vi "Julabo_Get_All_Values_subVI.vi"(4 "Reset / Default (T: Both)":bool=TRUE, 6 "ID Query? (T: Yes)":bool=TRUE, 7 "Data Cluster In":T1={"Current DoE"=[], "SSI 1 Flow Rate"=0.0, "SSI 2 Flow Rate"=0.0, "FLOM 1 Flow Rate"=0.0, "FLOM 2 Flow Rate"=0.0, "Pumps Running?"=FALSE, "Boolean 2"=FALSE, "Boolean 3"=FALSE, "Boolean 4"=FALSE, "At Equilibrium?"=FALSE, "Script Running?"=FALSE, "Current Script Iteration"=0.0, "Total Script Iterations"=0.0, "FLOM Pumps VISA"="COM2", "SSI 1 Pump VISA"="COM76", "SSI 2 Pump VISA"="COM74", "Huber Unistat VISA"="COM1", "SSI 3 Pump VISA"="COM76", "SSI 4 Pump VISA"="COM76", "SSI 4 Flow Rate"=0.0, "SSI 3 Flow Rate"=0.0, "Flow Meter 1 Rate "=0.0, "Flow Meter 2 Rate"=0.0, "Flow Meter 3 Rate"=0.0, "Flow Meter 4 Rate"=0.0, "SSI 1 Flow Setpoint"=0.0, "SSI 2 Flow Setpoint"=0.0, "SSI 3 Flow Setpoint"=0.0, "SSI 4 Flow Setpoint"=0.0, "Temperature Setpoint"=0.0, "Flow meter 3 COM"=17, "Flow meter 5 COM"=18, "Flow meter 4 COM"=19, "Flow meter 2 COM"=16, "Flow meter 1 COM"=15, "Unit"=enum."PSI", "Pressure COM"="COM6", "Julabo Setpoint"=0.0, "Julabo Control"=enum."Internal", "Overtemp"=50.0, "Subtemp"=-20.0, "HeatMax"=50, "CoolMax"=-100, "InternMax"=50.0, "InternMin"=0.0, "Upper Bandlimit"=100.0, "Lower Bandlimit"=0.0, "Julabo CF41 VISA"="COM3", "Xp (0.6K) Int"=0.6, "Tn (3s) Int"=3, "Tv (0s) Int"=0, "Dynamic (0: aperiodic) Int"=enum."aperiodic", "Xp (0.6K) Ext"=0.6, "Tn (3s) Ext"=3, "Tv (0s) Ext"=0, "XpU (0.6K) Ext"=0.6} {"XpU (0.6K) Ext" min=0.1 max=99.9; "Tv (0s) Ext" max=999; "Tn (3s) Ext" min=3 max=9999; "Xp (0.6K) Ext" min=0.1 max=99.9; "Tv (0s) Int" max=999; "Tn (3s) Int" min=3 max=9999; "Xp (0.6K) Int" min=0.1 max=99.9; "Lower Bandlimit" min=0.0 max=200.0; "Upper Bandlimit" min=0.0 max=200.0; "InternMin" format="%.2f"; "InternMax" format="%.2f"; "CoolMax" min=-100 max=0; "HeatMax" max=100; "Subtemp" format="%.2f"; "Overtemp" format="%.2f"; "Julabo Setpoint" format="%.2f"; "Current DoE" format="%0.3f"}, 9 "Serial Configuration":T2={"Baud Rate"=4800, "Parity"=2, "Data Bits"=7, "Stop Bits"=10, "Flow Control"=2} {"Flow Control" items=["None", "XON/XOFF", "RTS/CTS", "XON/XOFF & RTS/CTS", "DTR/DSR", "XON/XOFF & DTR/DSR"]; "Stop Bits" items=["1.0"=10, "1.5"=15, "2.0"=20]; "Data Bits" items=["7"=7, "8"=8]; "Parity" items=["None", "Odd", "Even", "Mark", "Space"]; "Baud Rate" items=["300"=300, "600"=600, "1200"=1200, "2400"=2400, "4800"=4800, "9600"=9600, "19200"=19200]}, 10 "RS485-Address (128: RS232)":u32=128, 11 "VISA Refnum in":refnum<visa-resource-name>="COM3") -> (0 "error out":errorcluster, 2 "Setpointindex":enum16{"Setpoint 1", "Setpoint 2", "Setpoint 3"}(ring), 5 "Data Cluster Out":T1={"Current DoE"=[], "SSI 1 Flow Rate"=0.0, "SSI 2 Flow Rate"=0.0, "FLOM 1 Flow Rate"=0.0, "FLOM 2 Flow Rate"=0.0, "Pumps Running?"=FALSE, "Boolean 2"=FALSE, "Boolean 3"=FALSE, "Boolean 4"=FALSE, "At Equilibrium?"=FALSE, "Script Running?"=FALSE, "Current Script Iteration"=0.0, "Total Script Iterations"=0.0, "FLOM Pumps VISA"="COM2", "SSI 1 Pump VISA"="COM76", "SSI 2 Pump VISA"="COM74", "Huber Unistat VISA"="COM1", "SSI 3 Pump VISA"="COM76", "SSI 4 Pump VISA"="COM76", "SSI 4 Flow Rate"=0.0, "SSI 3 Flow Rate"=0.0, "Flow Meter 1 Rate "=0.0, "Flow Meter 2 Rate"=0.0, "Flow Meter 3 Rate"=0.0, "Flow Meter 4 Rate"=0.0, "SSI 1 Flow Setpoint"=0.0, "SSI 2 Flow Setpoint"=0.0, "SSI 3 Flow Setpoint"=0.0, "SSI 4 Flow Setpoint"=0.0, "Temperature Setpoint"=0.0, "Flow meter 3 COM"=17, "Flow meter 5 COM"=18, "Flow meter 4 COM"=19, "Flow meter 2 COM"=16, "Flow meter 1 COM"=15, "Unit"=enum."PSI", "Pressure COM"="COM6", "Julabo Setpoint"=0.0, "Julabo Control"=enum."Internal", "Overtemp"=50.0, "Subtemp"=-20.0, "HeatMax"=50, "CoolMax"=-100, "InternMax"=50.0, "InternMin"=0.0, "Upper Bandlimit"=100.0, "Lower Bandlimit"=0.0, "Julabo CF41 VISA"="COM3", "Xp (0.6K) Int"=0.6, "Tn (3s) Int"=3, "Tv (0s) Int"=0, "Dynamic (0: aperiodic) Int"=enum."aperiodic", "Xp (0.6K) Ext"=0.6, "Tn (3s) Ext"=3, "Tv (0s) Ext"=0, "XpU (0.6K) Ext"=0.6} {"XpU (0.6K) Ext" min=0.1 max=99.9; "Tv (0s) Ext" max=999; "Tn (3s) Ext" min=3 max=9999; "Xp (0.6K) Ext" min=0.1 max=99.9; "Tv (0s) Int" max=999; "Tn (3s) Int" min=3 max=9999; "Xp (0.6K) Int" min=0.1 max=99.9; "Lower Bandlimit" min=0.0 max=200.0; "Upper Bandlimit" min=0.0 max=200.0; "InternMin" format="%.2f"; "InternMax" format="%.2f"; "CoolMax" min=-100 max=0; "HeatMax" max=100; "Subtemp" format="%.2f"; "Overtemp" format="%.2f"; "Julabo Setpoint" format="%.2f"; "Current DoE" format="%0.3f"})   [LabVIEW 2015, in "JULABO DeviceDriver.lvlib"]
uses:
  <instrlib>/JULABO DeviceDriver/JULABO DeviceDriver.lvlib
  <instrlib>/JULABO DeviceDriver/Examples/Julabo Serial Control.ctl
  --Controls and TypeDefs--/DoE_Control_Cluster.ctl
panel:
  # "Julabo"
  # "Limits"
  # "PID Control Parameters"
  # "Julabo"
  # "Limits"
  # "PID Control Parameters"
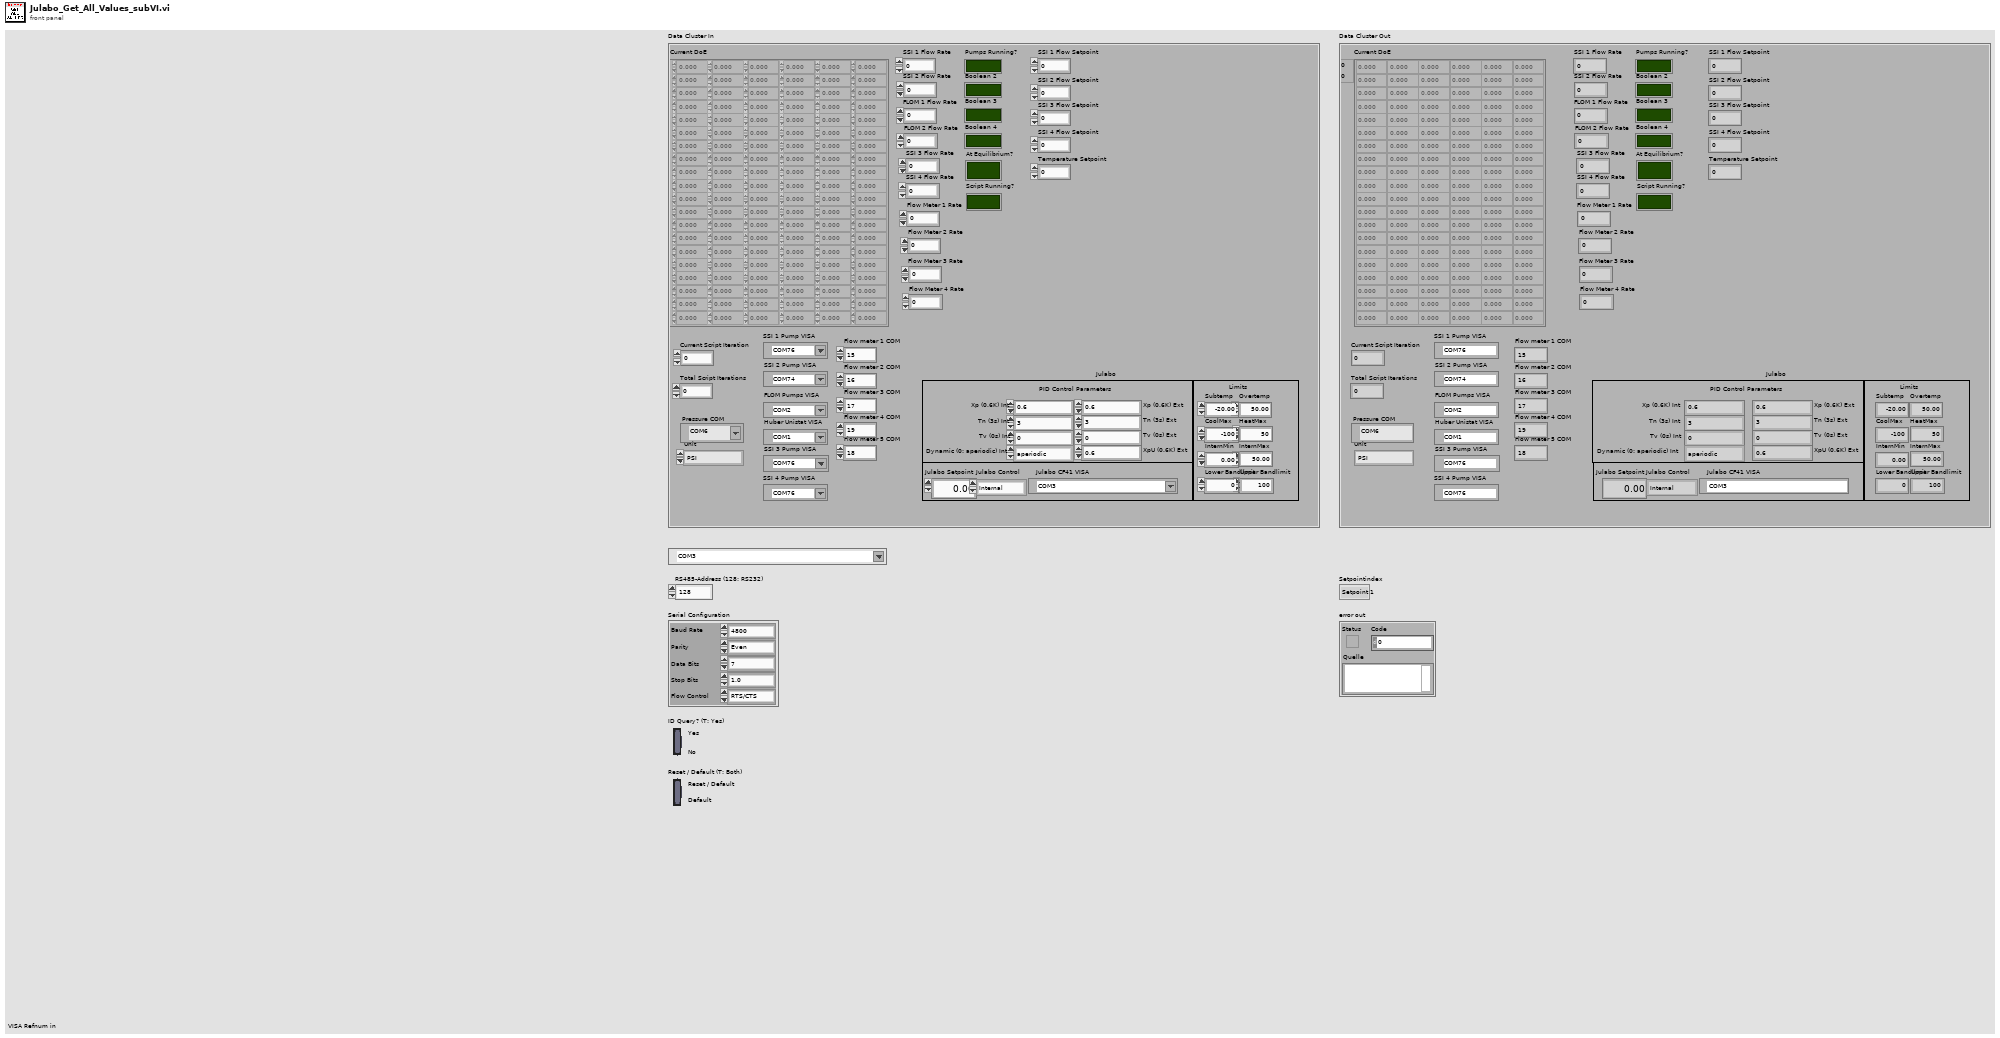
[diagram p1: front panel]
types:
  T1 = typedef "DoE_Control_Cluster.ctl" = cluster{"Current DoE":dbl[][], "SSI 1 Flow Rate":dbl, "SSI 2 Flow Rate":dbl, "FLOM 1 Flow Rate":dbl, "FLOM 2 Flow Rate":dbl, "Pumps Running?":bool, "Boolean 2":bool, "Boolean 3":bool, "Boolean 4":bool, "At Equilibrium?":bool, "Script Running?":bool, "Current Script Iteration":dbl, "Total Script Iterations":dbl, "FLOM Pumps VISA":refnum<visa-resource-name>, "SSI 1 Pump VISA":refnum<visa-resource-name>, "SSI 2 Pump VISA":refnum<visa-resource-name>, "Huber Unistat VISA":refnum<visa-resource-name>, "SSI 3 Pump VISA":refnum<visa-resource-name>, "SSI 4 Pump VISA":refnum<visa-resource-name>, "SSI 4 Flow Rate":dbl, "SSI 3 Flow Rate":dbl, "Flow Meter 1 Rate ":dbl, "Flow Meter 2 Rate":dbl, "Flow Meter 3 Rate":dbl, "Flow Meter 4 Rate":dbl, "SSI 1 Flow Setpoint":dbl, "SSI 2 Flow Setpoint":dbl, "SSI 3 Flow Setpoint":dbl, "SSI 4 Flow Setpoint":dbl, "Temperature Setpoint":dbl, "Flow meter 3 COM":u16, "Flow meter 5 COM":u16, "Flow meter 4 COM":u16, "Flow meter 2 COM":u16, "Flow meter 1 COM":u16, "Unit":enum16{"PSI", "Bar", "cm H2O", "ft H2O", "hectoPascal", "in Hg", "in H2O", "kiloPascal", "milliBar", "mmHg", "MegaPascal", "Numeric Pressure"}, "Pressure COM":refnum<visa-resource-name>, "Julabo Setpoint":dbl, "Julabo Control":enum16{"Internal", "External"}, "Overtemp":dbl, "Subtemp":dbl, "HeatMax":u8, "CoolMax":i8, "InternMax":dbl, "InternMin":dbl, "Upper Bandlimit":dbl, "Lower Bandlimit":dbl, "Julabo CF41 VISA":refnum<visa-resource-name>, "Xp (0.6K) Int":dbl, "Tn (3s) Int":u16, "Tv (0s) Int":u16, "Dynamic (0: aperiodic) Int":enum16{"aperiodic", "standard"}, "Xp (0.6K) Ext":dbl, "Tn (3s) Ext":u16, "Tv (0s) Ext":u16, "XpU (0.6K) Ext":dbl}
  T2 = typedef "Julabo Serial Control.ctl" = cluster{"Baud Rate":u32, "Parity":u16, "Data Bits":u16, "Stop Bits":u16, "Flow Control":u16}
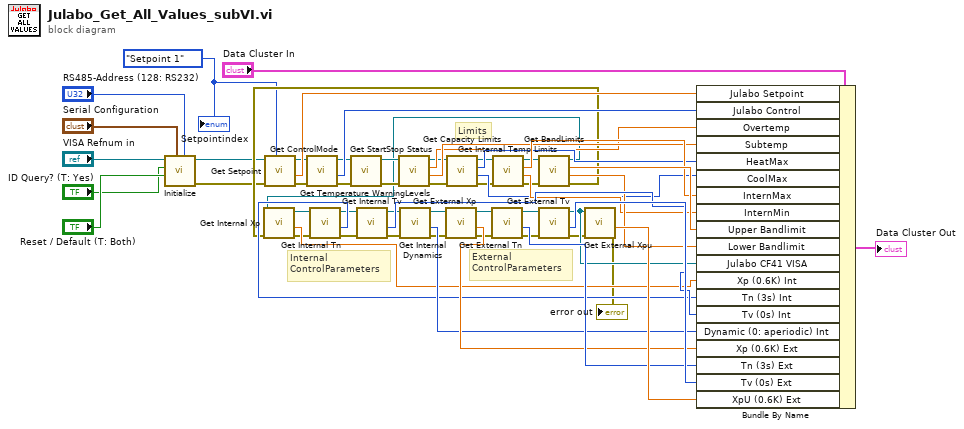
[diagram p0: block diagram]
diagram:
  w9 = enum16{"Setpoint 1", "Setpoint 2", "Setpoint 3"}."Setpoint 1" ("Setpointindex")
  # "External\nControlParameters"
  # "Internal\nControlParameters"
  # "Limits"
  n1 = call <instrlib>:"Initialize.vi"("RS485-Address (128: RS232)"="RS485-Address (128: RS232)", "Serial Configuration"="Serial Configuration", "Reset / Default (T: Both)"="Reset / Default (T: Both)", "ID Query? (T: Yes)"="ID Query? (T: Yes)", "VISA resource name"="VISA Refnum in") -> ("error out"=w8:errorcluster, "VISA resource name out"=w7:refnum<visa-resource-name>)  [unwired: 5 in]
  n2 = call <instrlib>:"Get Setpoint.vi"("Setpointindex"=w9, "error in (no error)"=w8, "VISA resource name"=w7) -> ("error out"=w38:errorcluster, "Setpoint (out)"=w39:dbl, "VISA resource name out"=w37:refnum<visa-resource-name>)  [unwired: 6 in]
  n3 = call <instrlib>:"Get ControlMode.vi"("error in"=w38, "VISA resource name in"=w37) -> ("error out"=w35:errorcluster, "Control (out)"=w40:enum16{"Internal", "External"}, "VISA resource name out"=w32:refnum<visa-resource-name>)  [unwired: 7 in]
  n4 = call <instrlib>:"Get StartStop Status.vi"("error in"=w35, "VISA resource name in"=w32) -> ("error out"=w36:errorcluster, "VISA resource name out"=w34:refnum<visa-resource-name>)  [unwired: 7 in, 1 out]
  n5 = call <instrlib>:"Get Temperature WarningLevels.vi"("error in (no error)"=w36, "VISA resource name"=w34) -> ("error out"=w14:errorcluster, "Subtemp (out)"=w42:dbl, "Overtemp (out)"=w41:dbl, "VISA resource name out"=w11:refnum<visa-resource-name>)  [unwired: 2 in]
  n6 = call <instrlib>:"Get Capacity Limits.vi"("error in (no error)"=w14, "VISA resource name"=w11) -> ("error out"=w15:errorcluster, "Maximum cooling capacity(out)"=w44:i8, "Maximum heating capacity(out)"=w43:u8, "VISA resource name out"=w12:refnum<visa-resource-name>)  [unwired: 2 in]
  n7 = call <instrlib>:"Get Internal Temp Limits.vi"("error in (no error)"=w15, "VISA resource name"=w12) -> ("error out"=w16:errorcluster, "IntMin (out)"=w46:dbl, "IntMax (out)"=w45:dbl, "VISA resource name out"=w13:refnum<visa-resource-name>)  [unwired: 2 in]
  n8 = call <instrlib>:"Get BandLimits.vi"("error in (no error)"=w16, "VISA resource name"=w13) -> ("error out"=w24:errorcluster, "LowerBand (out)"=w48:dbl, "UpperBand (out)"=w47:dbl, "VISA resource name out"=w23:refnum<visa-resource-name>)  [unwired: 2 in]
  n9 = call <instrlib>:"Get Internal Xp.vi"("error in"=w24, "VISA resource name in"=w23) -> ("error out"=w22:errorcluster, "InternalXp (out)"=w50:dbl, "VISA resource name out"=w21:refnum<visa-resource-name>)  [unwired: 7 in]
  n10 = call <instrlib>:"Get Internal Tn.vi"("error in"=w22, "VISA resource name in"=w21) -> ("error out"=w20:errorcluster, "InternalTn (out)"=w51:u16, "VISA resource name out"=w19:refnum<visa-resource-name>)  [unwired: 7 in]
  n11 = call <instrlib>:"Get Internal Tv.vi"("error in"=w20, "VISA resource name in"=w19) -> ("error out"=w18:errorcluster, "InternalTv (out)"=w52:u16, "VISA resource name out"=w17:refnum<visa-resource-name>)  [unwired: 7 in]
  n12 = call <instrlib>:"Get Internal Dynamics.vi"("error in"=w18, "VISA resource name in"=w17) -> ("error out"=w29:errorcluster, "Dynamic (out)"=w53:enum16{"aperiodic", "standard"}, "VISA resource name out"=w30:refnum<visa-resource-name>)  [unwired: 7 in]
  n13 = call <instrlib>:"Get External Xp.vi"("error in"=w29, "VISA resource name in"=w30) -> ("error out"=w28:errorcluster, "ExternalXp (out)"=w54:dbl, "VISA resource name out"=w31:refnum<visa-resource-name>)  [unwired: 7 in]
  n14 = call <instrlib>:"Get External Tn.vi"("error in"=w28, "VISA resource name in"=w31) -> ("error out"=w25:errorcluster, "ExternalTn (out)"=w55:u16, "VISA resource name out"=w26:refnum<visa-resource-name>)  [unwired: 7 in]
  n15 = call <instrlib>:"Get External Tv.vi"("error in"=w25, "VISA resource name in"=w26) -> ("error out"=w27:errorcluster, "ExternalTv (out)"=w56:u16, "VISA resource name out"=w49:refnum<visa-resource-name>)  [unwired: 7 in]
  n16 = call <instrlib>:"Get External Xpu.vi"("error in"=w27, "VISA resource name in"=w49) -> ("error out"=→"error out":errorcluster, "ExternalXpu (out)"=w57:dbl)  [unwired: 7 in, 1 out]
  n17 = Bundle By Name(cluster="Data Cluster In", "Julabo Setpoint"=w39, "Julabo Control"=w40, "Overtemp"=w41, "Subtemp"=w42, "HeatMax"=w43, "CoolMax"=w44, "InternMax"=w45, "InternMin"=w46, "Upper Bandlimit"=w47, "Lower Bandlimit"=w48, "Julabo CF41 VISA"=w49, "Xp (0.6K) Int"=w50, "Tn (3s) Int"=w51, "Tv (0s) Int"=w52, "Dynamic (0: aperiodic) Int"=w53, "Xp (0.6K) Ext"=w54, "Tn (3s) Ext"=w55, "Tv (0s) Ext"=w56, "XpU (0.6K) Ext"=w57) -> (→"Data Cluster Out":T1)
  "Setpointindex" <- w9
